vi "PathPlanner_Cmd_Follow_Internal_Sample.vi"(4 "PassthroughTime_SEC":dbl, 5 "Extra Time Sec":dbl, 6 "Reset In":bool, 8 "Position Error M":dbl, 9 "Current Pose SI":T20 {"ROTATION"."SIN" format="%13.4f"; "ROTATION"."COS" format="%13.4f"; "ROTATION"."VALUE" format="%13.4f"; "TRANSLATION"."Y" format="%14.3f"; "TRANSLATION"."X" format="%14.3f"}, 10 "CurrentChassisSpeeds":T21 {"vOmega" format="%10.3f"; "vY" format="%10.3f"; "vX" format="%10.3f"}, 11 "RePlannedPath in":T11={"Reversed"=FALSE, "RotationTargets"=[], "ConstraintZones"=[], "EventMarkers"=[], "GlobalConstraints"={"MaxVelocityMps;"=0.0, "MaxAccelerationMpsSq;"=0.0, "MaxAngularVelRadPsEc;"=0.0, "MaxAngularAccRadPSecSq"=0.0, "Exists"=FALSE, "Unlimited"=FALSE, "NominalVoltageVolts"=12.0}, "GoalEndState"={"VelocityMPS"=0.0, "Rotation"={"VALUE"=0.0, "COS"=0.0, "SIN"=0.0}}, "AllPoints"=[], "Name"="", "Waypoints"=[], "PointTowardsZones"=[], "IdealStartingState"={"VelocityMPS"=0.0, "Rotation"={"VALUE"=0.0, "COS"=0.0, "SIN"=0.0}}, "IsChoreoPath"=FALSE, "PreventFlipping"=FALSE} {"IdealStartingState"."Rotation"."SIN" format="%13.4f"; "IdealStartingState"."Rotation"."COS" format="%13.4f"; "IdealStartingState"."Rotation"."VALUE" format="%13.4f"; "PointTowardsZones"."TargetPosition"."Y" format="%14.3f"; "PointTowardsZones"."TargetPosition"."X" format="%14.3f"; "PointTowardsZones"."RotationOffset"."SIN" format="%13.4f"; "PointTowardsZones"."RotationOffset"."COS" format="%13.4f"; "PointTowardsZones"."RotationOffset"."VALUE" format="%13.4f"; "Waypoints"."nextControl"."Y" format="%14.3f"; "Waypoints"."nextControl"."X" format="%14.3f"; "Waypoints"."anchor"."Y" format="%14.3f"; "Waypoints"."anchor"."X" format="%14.3f"; "Waypoints"."prevControl"."Y" format="%14.3f"; "Waypoints"."prevControl"."X" format="%14.3f"; "AllPoints"."RotationTarget"."rotation"."SIN" format="%13.4f"; "AllPoints"."RotationTarget"."rotation"."COS" format="%13.4f"; "AllPoints"."RotationTarget"."rotation"."VALUE" format="%13.4f"; "AllPoints"."Position"."Y" format="%14.3f"; "AllPoints"."Position"."X" format="%14.3f"; "GoalEndState"."Rotation"."SIN" format="%13.4f"; "GoalEndState"."Rotation"."COS" format="%13.4f"; "GoalEndState"."Rotation"."VALUE" format="%13.4f"; "RotationTargets"."rotation"."SIN" format="%13.4f"; "RotationTargets"."rotation"."COS" format="%13.4f"; "RotationTargets"."rotation"."VALUE" format="%13.4f"}) -> (0 "Traj End Status":T6, 1 "Trajectory State":T7={"TimeSeconds"=0.0, "VelocityMPS"=0.0, "AccerationMpsSq"=0.0, "HeadingAngularVelRadPerSec"=0.0, "PositionMeters"={"X"=0.0, "Y"=0.0}, "Heading"={"VALUE"=0.0, "COS"=1.0, "SIN"=0.0}, "TargetHolonomicRotation"={"VALUE"=0.0, "COS"=1.0, "SIN"=0.0}, "CurvatureRadPerMeter"=0.0, "PathPlannerConstraints"={"MaxVelocityMps;"=0.0, "MaxAccelerationMpsSq;"=0.0, "MaxAngularVelRadPsEc;"=0.0, "MaxAngularAccRadPSecSq"=0.0, "Exists"=FALSE, "Unlimited"=FALSE, "NominalVoltageVolts"=12.0}, "DeltaPos"=0.0, "WaypointRelPos"=0.0} {"TargetHolonomicRotation"."SIN" format="%13.4f"; "TargetHolonomicRotation"."COS" format="%13.4f"; "TargetHolonomicRotation"."VALUE" format="%13.4f"; "Heading"."SIN" format="%13.4f"; "Heading"."COS" format="%13.4f"; "Heading"."VALUE" format="%13.4f"; "PositionMeters"."Y" format="%14.3f"; "PositionMeters"."X" format="%14.3f"}, 2 "Reset Controller":bool, 3 "PathPlannerTrajectoryEvents":T1)   [LabVIEW 2019, in "PathPlanner24.lvlib"]
doc: "This is an internal function. It is not to be called by end users."
uses:
  PathPlanner24.lvlib
  <vilib>/Rock Robotics/WPI/ThirdParty/JAS_Junk/TrajLib/Trajectory_Library.lvlib
  <vilib>/Rock Robotics/WPI/ThirdParty/JAS_Junk/TrajLib/TypeDef/TRANSLATION2D.ctl
  <vilib>/Rock Robotics/WPI/ThirdParty/JAS_Junk/TrajLib/TypeDef/ROTATION2D.ctl
  TypeDef/PathPlannerPathConstraints.ctl
  <vilib>/Rock Robotics/WPI/ThirdParty/JAS_Junk/TrajLib/TypeDef/CHASSIS_SPEEDS.ctl
  TypeDef/PathPlannerRotationTarget.ctl
  TypeDef/PathPlannerConstraintsZone.ctl
  ENum/PathPlanner_TrajectoryEvent_Type_ENUM.ctl
  TypeDef/PathPlannerCommandUtil.ctl
  TypeDef/PathPlannerEventMarker.ctl
  TypeDef/PathPlannerGoalEndState.ctl
  TypeDef/PathPlannerPathPoint.ctl
  TypeDef/PathPlannerPath.ctl
  <vilib>/Rock Robotics/WPI/ThirdParty/JAS_Junk/TrajLib/TypeDef/POSE2D.ctl
  TypeDef/PathPlannerTrajectoryState.ctl
  TypeDef/PathPlannerTrajectoryEvent.ctl
  TypeDef/PathPlannerTrajectoryEvents.ctl
  TypeDef/PathPlannerWaypoint.ctl
  TypeDef/PathPlannerPointTowardsZone.ctl
  TypeDef/PathPlannerIdealStartingState.ctl
  ENum/PathPlanner_CommandUtil_Type_ENUM.ctl
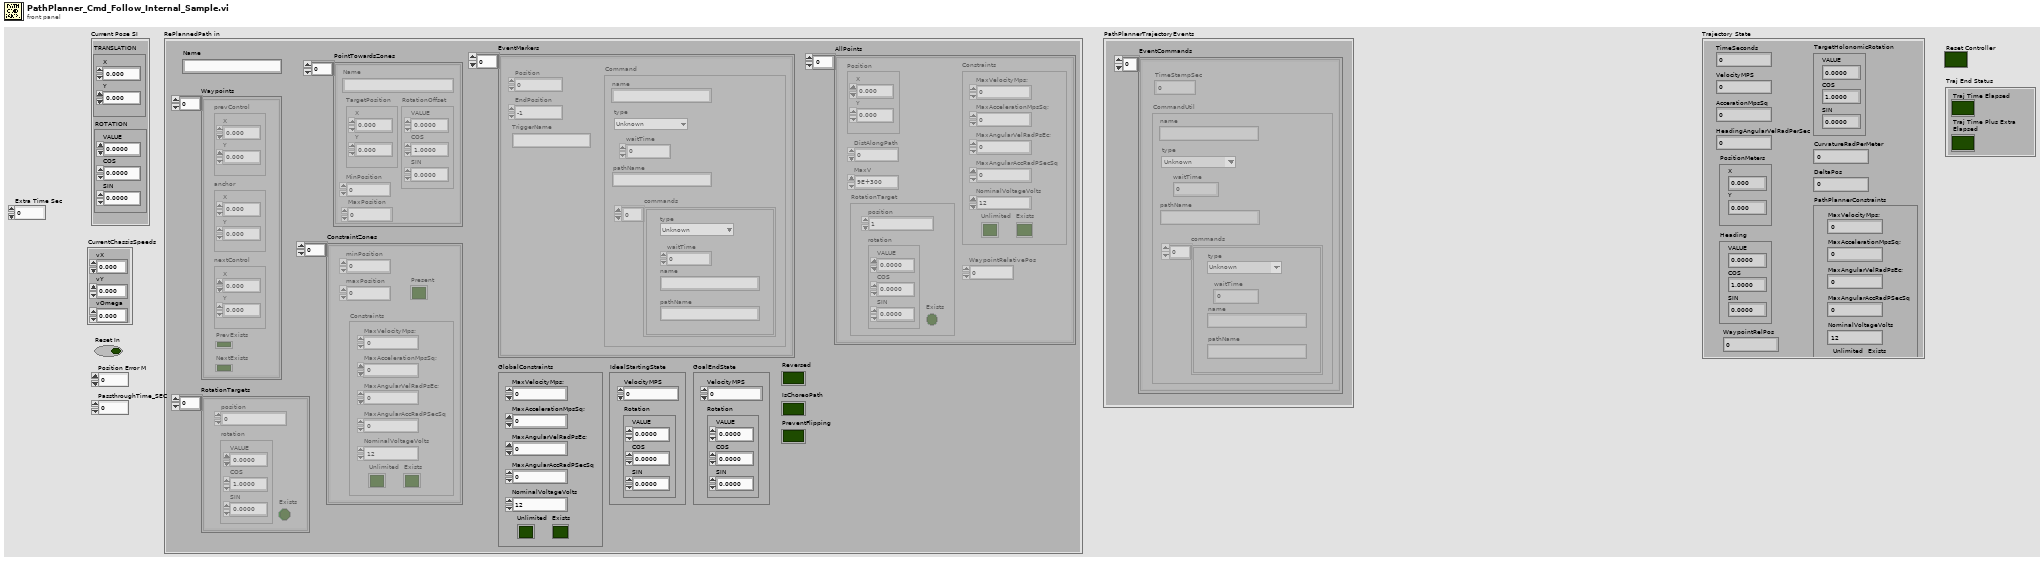
[diagram p1: front panel]
types:
  T1 = typedef "PathPlanner24.lvlib/PathPlannerTrajectoryEvents.ctl" = cluster{"EventCommands":T2[]}
  T2 = typedef "PathPlanner24.lvlib/PathPlannerTrajectoryEvent.ctl" = cluster{"TimeStampSec":dbl, "CommandUtil":T3}
  T3 = typedef "PathPlanner24.lvlib/PathPlannerCommandUtil.ctl" = cluster{"waitTime":dbl, "name":string, "pathName":string, "commands":cluster{"type":T4, "waitTime":dbl, "name":string, "pathName":string}[], "type":T5}
  T4 = typedef "PathPlanner24.lvlib/PathPlanner_TrajectoryEvent_Type_ENUM.ctl" = enum16{"Unknown", "Wait", "Named", "Path", "Sequential", "Parallel", "Race", "Deadline", "PointTowardsZoneEnter", "PointTowardsZoneExit", "TriggerEventStart", "TriggerEventStop", "TriggerEventOneshot"}
  T5 = typedef "PathPlanner24.lvlib/PathPlanner_CommandUtil_Type_ENUM.ctl" = enum16{"Unknown", "Wait", "Named", "Path", "Sequential", "Parallel", "Race", "Deadline"}
  T6 = cluster{"Traj Time Plus Extra\nElapsed":bool, "Traj Time Elapsed":bool}
  T7 = typedef "PathPlanner24.lvlib/PathPlannerTrajectoryState.ctl" = cluster{"TimeSeconds":dbl, "VelocityMPS":dbl, "AccerationMpsSq":dbl, "HeadingAngularVelRadPerSec":dbl, "PositionMeters":T8, "Heading":T9, "TargetHolonomicRotation":T9, "CurvatureRadPerMeter":dbl, "PathPlannerConstraints":T10, "DeltaPos":dbl, "WaypointRelPos":dbl}
  T8 = typedef "Trajectory_Library.lvlib/TRANSLATION2D.ctl" = cluster{"X":dbl, "Y":dbl}
  T9 = typedef "Trajectory_Library.lvlib/ROTATION2D.ctl" = cluster{"VALUE":dbl, "COS":dbl, "SIN":dbl}
  T10 = typedef "PathPlanner24.lvlib/PathPlannerPathConstraints.ctl" = cluster{"MaxVelocityMps;":dbl, "MaxAccelerationMpsSq;":dbl, "MaxAngularVelRadPsEc;":dbl, "MaxAngularAccRadPSecSq":dbl, "Exists":bool, "Unlimited":bool, "NominalVoltageVolts":dbl}
  T11 = typedef "PathPlanner24.lvlib/PathPlannerPath.ctl" = cluster{"Reversed":bool, "RotationTargets":T12[], "ConstraintZones":T13[], "EventMarkers":T14[], "GlobalConstraints":T10, "GoalEndState":T15, "AllPoints":T16[], "Name":string, "Waypoints":T17[], "PointTowardsZones":T18[], "IdealStartingState":T19, "IsChoreoPath":bool, "PreventFlipping":bool}
  T12 = typedef "PathPlanner24.lvlib/PathPlannerRotationTarget.ctl" = cluster{"position":dbl, "rotation":T9, "Exists":bool}
  T13 = typedef "PathPlanner24.lvlib/PathPlannerConstraintsZone.ctl" = cluster{"minPosition":dbl, "maxPosition":dbl, "Constraints":T10, "Present":bool}
  T14 = typedef "PathPlanner24.lvlib/PathPlannerEventMarker.ctl" = cluster{"Position":dbl, "Command":T3, "TriggerName":string, "EndPosition":dbl}
  T15 = typedef "PathPlanner24.lvlib/PathPlannerGoalEndState.ctl" = cluster{"VelocityMPS":dbl, "Rotation":T9}
  T16 = typedef "PathPlanner24.lvlib/PathPlannerPathPoint.ctl" = cluster{"Position":T8, "DistAlongPath":dbl, "MaxV":dbl, "Constraints":T10, "RotationTarget":T12, "WaypointRelativePos":dbl}
  T17 = typedef "PathPlanner24.lvlib/PathPlannerWaypoint.ctl" = cluster{"prevControl":T8, "anchor":T8, "nextControl":T8, "PrevExists":bool, "NextExists":bool}
  T18 = typedef "PathPlanner24.lvlib/PathPlannerPointTowardsZone.ctl" = cluster{"RotationOffset":T9, "Name":string, "TargetPosition":T8, "MinPosition":dbl, "MaxPosition":dbl}
  T19 = typedef "PathPlanner24.lvlib/PathPlannerIdealStartingState.ctl" = cluster{"VelocityMPS":dbl, "Rotation":T9}
  T20 = typedef "Trajectory_Library.lvlib/POSE2D.ctl" = cluster{"TRANSLATION":T8, "ROTATION":T9}
  T21 = typedef "Trajectory_Library.lvlib/CHASSIS_SPEEDS.ctl" = cluster{"vX":dbl, "vY":dbl, "vOmega":dbl}
  T22 = typedef "PathPlanner24.lvlib/PathPlannerTrajectory.ctl" = cluster{"States":T7[]}
  T23 = typedef "Trajectory_Library.lvlib/TIMER.ctl" = cluster{"StartTime":dbl, "Accumulated TIme":dbl, "Running":bool, "semaphore":T24}
  T24 = typedef "Semaphore RefNum" = refnum<k1>
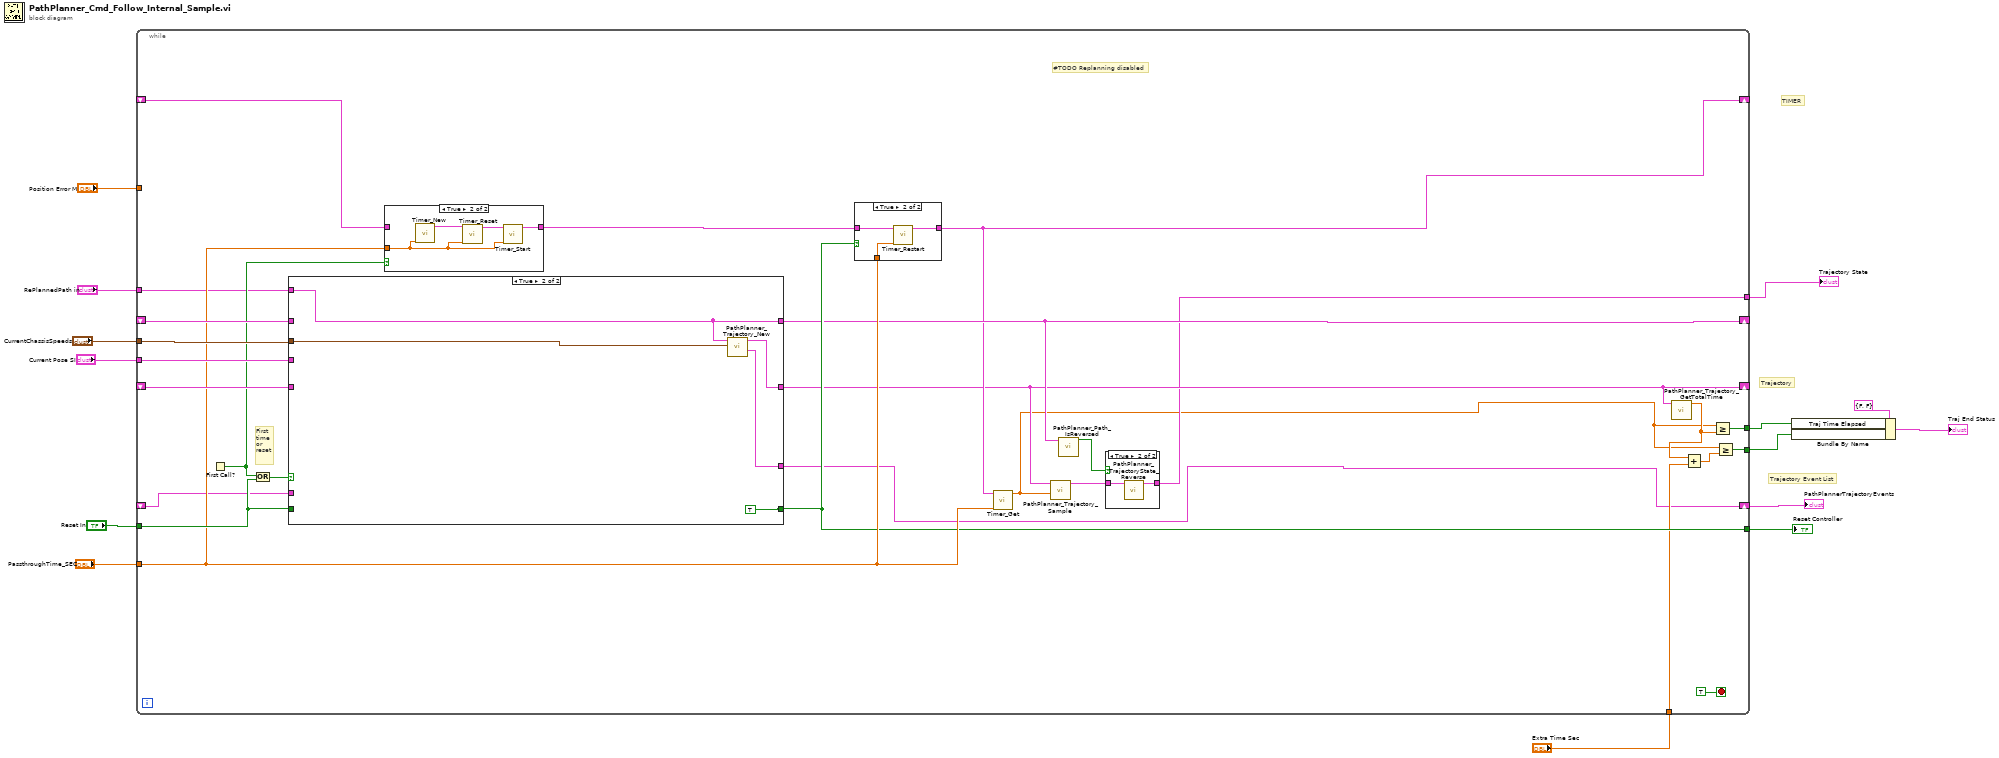
[diagram p0: block diagram]
diagram:
  # "Trajectory Event List"
  # "TIMER"
  # "Trajectory"
  n1 = while {
    tunnel: "CurrentChassisSpeeds" -> [w36]
    tunnel: "Current Pose SI" -> [w35]
    shift-right: [w26] -> _
    shift-left: _ -> [w41]
    shift-right: [w29] -> _
    shift-left: _ -> [w40]
    tunnel: "Reset In" -> [w39]
    tunnel: [w30] -> w12
    tunnel: [w19] -> w10
    tunnel: "PassthroughTime_SEC" -> [w32]
    shift-right: [w28] -> _
    shift-left: _ -> [w33]
    tunnel: "Position Error M" -> [_]
    tunnel: [w25] -> w5
    tunnel: [w22] -> w4
    tunnel: "Extra Time Sec" -> [w21]
    shift-right: [w17] -> w1
    shift-left: _ -> [w16]
    tunnel: "RePlannedPath in" -> [w15]
    stop <- TRUE stop-if-true
    # "#TODO Replanning disabled"
    # "First\ntime\nor \nreset"
    n2 = First Call?() -> (First Call?: T/F=w27:bool)
    n3 = Or(x=w27, y=w39) -> (x .or. y?=w38:bool)
    n4 = case shown="True" w38 {
      tunnel: w40 -> [w56 _]
      tunnel: w36 -> [_ w62]
      tunnel: [w55 w61] -> w26
      tunnel: w35 -> [_ _]
      tunnel: [w56 w60] -> w29
      tunnel: w41 -> [w55 _]
      tunnel: w39 -> [w57 _]
      tunnel: [w57 TRUE] -> w30
      tunnel: [w54 w58] -> w17
      tunnel: w16 -> [w54 _]
      tunnel: w15 -> [_ w60]
      frame False {
      }
      frame True {
        n5 = call "PathPlanner_Trajectory_New.vi"("StartingSpeeds"=w62, "Path"=w60) -> ("PathPlannerTrajectoryEvents"=w58:T1, "PathPlannerTrajectory"=w61:T22)  [unwired: 8 in]
      }
    }
    n6 = case shown="True" w27 {
      tunnel: w32 -> [_ w51]
      tunnel: [w49 w50] -> w34
      tunnel: w33 -> [w49 _]
      frame False {
      }
      frame True {
        n7 = call <vilib>:"Timer_New.vi"("Pass_Through_Time"=w51) -> ("TIMER"=w53:T23)  [unwired: 10 in]
        n8 = call <vilib>:"Timer_Reset.vi"("Pass_Through_Time"=w51, "in TIMER"=w53) -> ("out TIMER"=w52:T23)  [unwired: 9 in]
        n9 = call <vilib>:"Timer_Start.vi"("Pass_Through_Time"=w51, "in Timer"=w52) -> ("out Timer"=w50:T23)  [unwired: 9 in]
      }
    }
    n10 = case shown="True" w30 {
      tunnel: w34 -> [w42 w45]
      tunnel: [w42 w44] -> w28
      tunnel: w32 -> [_ w43]
      frame False {
      }
      frame True {
        n11 = call <vilib>:"Timer_Restart.vi"("Pass_Through_Time"=w43, "in Timer"=w45) -> ("out Timer"=w44:T23)  [unwired: 9 in]
      }
    }
    n12 = call <vilib>:"Timer_Get.vi"("Pass_Through_Time"=w32, "TIMER"=w28) -> ("CurrentTImer"=w18:dbl)  [unwired: 9 in]
    n13 = call "PathPlanner_Trajectory_Sample.vi"("Time"=w18, "PathPlannerTrajectory"=w26) -> ("PathPlannerState"=w31:T7)  [unwired: 9 in]
    n14 = call "PathPlanner_Path_IsReversed.vi"("PathPlannerPath"=w29) -> ("Reversed"=w20:bool)  [unwired: 10 in]
    n15 = case shown="True" w20 {
      tunnel: w31 -> [w46 w48]
      tunnel: [w46 w47] -> w19
      frame False {
      }
      frame True {
        n16 = call "PathPlanner_TrajectoryState_Reverse.vi"("PathPlannerState"=w48) -> ("Reversed State"=w47:T7)  [unwired: 10 in]
      }
    }
    n17 = call "PathPlanner_Trajectory_GetTotalTime.vi"("PathPlannerTrajectory"=w26) -> ("TotalTimeSeconds"=w23:dbl)  [unwired: 10 in]
    n18 = Add(x=w23, y=w21) -> (x+y=w24:dbl)
    n19 = Greater Or Equal?(x=w18, y=w23) -> (x >= y?=w25:bool)
    n20 = Greater Or Equal?(x=w18, y=w24) -> (x >= y?=w22:bool)
  }
  "Reset Controller" <- w12
  "Trajectory State" <- w10
  "PathPlannerTrajectoryEvents" <- w1
  n21 = Bundle By Name(cluster=T6 {"Traj Time Plus Extra\nElapsed"=FALSE, "Traj Time Elapsed"=FALSE} ("Traj End Status"), "Traj Time Elapsed"=w5, "Traj Time Plus Extra\nElapsed"=w4) -> (→"Traj End Status":T6)
